vi "Simflight.vi"() -> ()   [LabVIEW 2014]
uses:
  subvis/state space loop data.ctl
  <vilib>/addons/Control Design/_Model Construction/Data Typedefs.llb/CD MIMO Time Response Data.ctl
  <vilib>/addons/Control Design/_Model Construction/Data Typedefs.llb/CD Plot Types Enum.ctl
  <vilib>/Utility/miscctls.llb/LV3DPointTypeDef.ctl
  <vilib>/Analysis/baseanly.llb/Real Outer Product.vi
  <vilib>/Analysis/Matrix/Numeric/Subtract/Subtract - RM,RM.vi
  <vilib>/addons/Control Design/_Model Construction/Model Creation.llb/Model Creation SubVI/cd_Create State Space Model.vi
  subvis/Data Xfer/subvis/Curcular Buffer Data History.vi
  <vilib>/Utility/inputDevices.llb/joystickAcquire.vi
  <vilib>/addons/Control Design/_Time Response Analysis/Time Response.llb/Time Response subVI/cd_Linear Simulation (State-Space).vi
  <vilib>/express/express arith-compare/Formula/XNode/ExpressFormulaBlockNode.xnode
  <vilib>/addons/Control Design/_Model Construction/NI_LinSys_Model Creation.lvlib
  <vilib>/addons/Control Design/_Time Response Analysis/NI_CD_Time Response.lvlib
  <vilib>/addons/Control Design/_Model Construction/NI_LinSys_Data Typedefs.lvlib
  subvis/attitude indicator/lv-attitudecontrol.lvlib
  <vilib>/Analysis/NI_AALBase.lvlib
  <vilib>/Analysis/Matrix/NI_Matrix.lvlib
panel:
  in  "device index":i32=2
  out "altitude 3":T1(graph)
  out "altitude 2":T1(graph)
  out "altitude":T1(graph)
  in  "elevator gain":dbl
  in  "aileron gain":dbl
  in  "rudder gain":dbl
  out "plot":T1(graph)
  in  "Aircraft":string="CDR"
  in  "Attitude Indicator":refnum<vi>(3d-picture)
  out "Airspeed (ft/s)":dbl(knob)=74.91519927978516 scale=0.0..80.0 scale format="%#.4f"
  out "motor (BHP)":cluster{dbl, dbl}(slide) scale=0.0..0.4
  out "ground track":cluster{"Time Stamp":dbl, "Data Value":dbl}[](graph)
  out "roll":dbl(slide) scale=-90.0..90.0
  out "pitch":dbl(slide) scale=-90.0..90.0
  out "rudder":cluster{dbl, dbl}(slide) scale=-25.0..25.0
  out "aileron":cluster{dbl, dbl}(slide) scale=-25.0..25.0
  out "elevator":cluster{dbl, dbl}(slide) scale=-35.0..35.0
  out "Heading":T2(graph)={"X"=[{"Y"=[21.620706805998168, 20.15124367946963, 12.465582235692763, 7.946576972490323, 11.656565240893995, 3.970903792227472, 5.440366929130449, 13.126028372052978, 19.003880895383112, 16.244982298473555, 16.832767550897515, 24.922937499080067, 24.33515224168201, 19.81289788882929, 13.93504536742159, 21.620706805998168], "Y"=[7.099604990531346, 5.077062500919932, 10.661022401488875, 5.291796067500631, 11.248807654089271, 16.832767550897515, 18.855310035128806, 13.271350139939326, 21.36152008350073, 25.220079209877188, 26.02909620777253, 20.151243679469633, 19.34222668734553, 20.773734831883043, 12.683564887248515, 7.099604990531346]}], "z"=[{"Y"=[15.0, 16.30733614, 17.60472267, 17.43107449, 17.60472267, 18.88228568, 20.13030215, 19.78828201, 20.13030215, 21.33927393, 22.5, 22.0, 22.5, 23.60364655, 24.64181415, 23.99902654, 24.64181415, 25.60660172, 26.49066665, 25.7246222, 26.49066665, 27.28728066, 27.99038106, 27.12435565, 27.99038106, 28.59461681, 29.09538931, 28.15569669, 29.09538931, 29.48888739, 29.7721163, 28.78730854, 29.7721163, 29.94292047, 30.0, 28.5, 30.0, 29.94292047, 29.7721163, 28.78730854, 29.7721163, 29.48888739, 29.09538931, 28.15569669, 29.09538931, 28.59461681, 27.99038106, 27.12435565, 27.99038106, 27.28728066, 26.49066665, 25.7246222, 26.49066665, 25.60660172, 24.64181415, 23.99902654, 24.64181415, 23.60364655, 22.5, 22.0, 22.5, 21.33927393, 20.13030215, 19.78828201, 20.13030215, 18.88228568, 17.60472267, 17.43107449, 17.60472267, 16.30733614, 15.0, 15.0, 15.0, 13.69266386, 12.39527733, 12.56892551, 12.39527733, 11.11771432, 9.86969785, 10.21171799, 9.86969785, 8.660726074, 7.5, 8.0, 7.5, 6.396353455, 5.358185855, 6.000973464, 5.358185855, 4.393398282, 3.509333353, 4.275377796, 3.509333353, 2.712719336, 2.009618943, 2.875644347, 2.009618943, 1.405383194, 0.904610688, 1.844303309, 0.904610688, 0.511112606, 0.227883705, 1.212691458, 0.227883705, 0.057079529, 0.0, 1.5, 0.0, 0.057079529, 0.227883705, 1.212691458, 0.227883705, 0.511112606, 0.904610688, 1.844303309, 0.904610688, 1.405383194, 2.009618943, 2.875644347, 2.009618943, 2.712719336, 3.509333353, 4.275377796, 3.509333353, 4.393398282, 5.358185855, 6.000973464, 5.358185855, 6.396353455, 7.5, 8.0, 7.5, 8.660726074, 9.86969785, 10.21171799, 9.86969785, 11.11771432, 12.39527733, 12.56892551, 12.39527733, 13.69266386, 15.0, 15.0], "Y"=[30.0, 29.94292047, 29.7721163, 28.78730854, 29.7721163, 29.48888739, 29.09538931, 28.15569669, 29.09538931, 28.59461681, 27.99038106, 27.12435565, 27.99038106, 27.28728066, 26.49066665, 25.7246222, 26.49066665, 25.60660172, 24.64181415, 23.99902654, 24.64181415, 23.60364655, 22.5, 22.0, 22.5, 21.33927393, 20.13030215, 19.78828201, 20.13030215, 18.88228568, 17.60472267, 17.43107449, 17.60472267, 16.30733614, 15.0, 15.0, 15.0, 13.69266386, 12.39527733, 12.56892551, 12.39527733, 11.11771432, 9.86969785, 10.21171799, 9.86969785, 8.660726074, 7.5, 8.0, 7.5, 6.396353455, 5.358185855, 6.000973464, 5.358185855, 4.393398282, 3.509333353, 4.275377796, 3.509333353, 2.712719336, 2.009618943, 2.875644347, 2.009618943, 1.405383194, 0.904610688, 1.844303309, 0.904610688, 0.511112606, 0.227883705, 1.212691458, 0.227883705, 0.057079529, 0.0, 1.5, 0.0, 0.057079529, 0.227883705, 1.212691458, 0.227883705, 0.511112606, 0.904610688, 1.844303309, 0.904610688, 1.405383194, 2.009618943, 2.875644347, 2.009618943, 2.712719336, 3.509333353, 4.275377796, 3.509333353, 4.393398282, 5.358185855, 6.000973464, 5.358185855, 6.396353455, 7.5, 8.0, 7.5, 8.660726074, 9.86969785, 10.21171799, 9.86969785, 11.11771432, 12.39527733, 12.56892551, 12.39527733, 13.69266386, 15.0, 15.0, 15.0, 16.30733614, 17.60472267, 17.43107449, 17.60472267, 18.88228568, 20.13030215, 19.78828201, 20.13030215, 21.33927393, 22.5, 22.0, 22.5, 23.60364655, 24.64181415, 23.99902654, 24.64181415, 25.60660172, 26.49066665, 25.7246222, 26.49066665, 27.28728066, 27.99038106, 27.12435565, 27.99038106, 28.59461681, 29.09538931, 28.15569669, 29.09538931, 29.48888739, 29.7721163, 28.78730854, 29.7721163, 29.94292047, 30.0, 28.5]}]}
  in  "visual":refnum<k7>(container) caption="3D 파라미터형 표면"
  in  "stop":bool
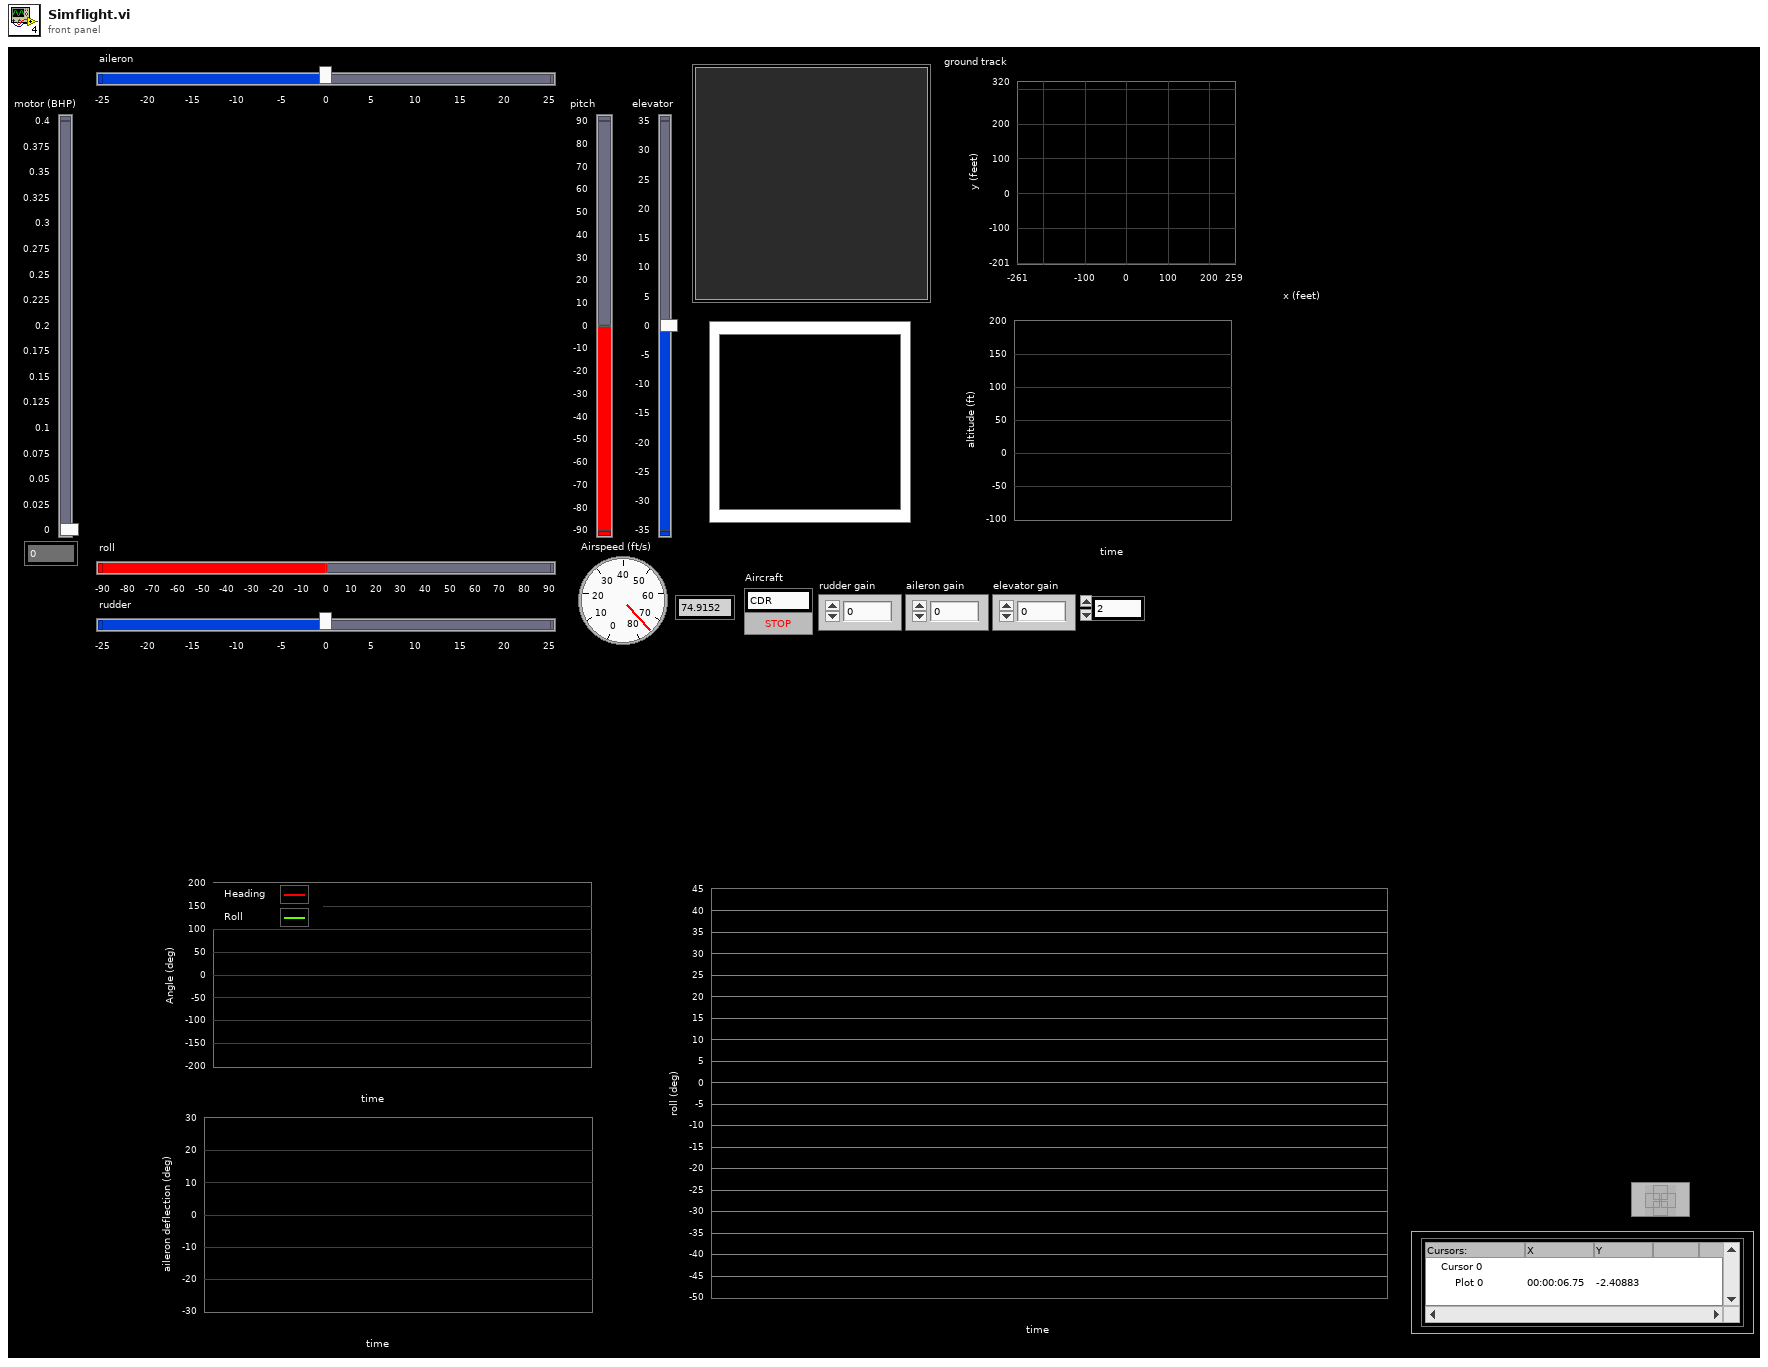
[diagram p1: front panel]
types:
  T1 = cluster{cluster{"Time Stamp":dbl, "Data Value":dbl}[]}[]
  T2 = cluster{"X":cluster{"Y":dbl[], "Y":dbl[]}[], "z":cluster{"Y":dbl[], "Y":dbl[]}[]}
  T3 = typedef "state space loop data.ctl" = cluster{"d_elevator (rad)":dbl, "d_rudder (rad)":dbl, "d_aileron (rad)":dbl, "d_motor (bhp)":dbl, "loop start (s)":dbl, "dT":dbl, "time now":dbl, "Sim Data":T4, "sim conditions":dbl[], "timestamp":dbl}
  T4 = typedef "NI_LinSys_Data Typedefs.lvlib/CD MIMO Time Response Data.ctl" = cluster{"Time":dbl[], "Outputs Data":dbl[][][], "States Data":dbl[][][], "plot type":T5}
  T5 = typedef "NI_LinSys_Data Typedefs.lvlib/CD Plot Types Enum.ctl" = enum16{"bode-magnitude", "bode-phase", "nichols", "nyquist", "singular values", "step", "impulse", "initial", "simulation", "nyquist with separation"}
  T6 = typedef "FlatEarth Inputs.ctl" = cluster{"a":dbl[][], "b":dbl[][], "c":dbl[][], "d":dbl[][], "du":dbl[][], "uIC":dbl[], "xIC":dbl[]}
  T7 = typedef "SIM INI.ctl" = cluster{"max_pwr":dbl, "max_rudder":dbl, "max_aileron":dbl, "max_elevator":dbl, "max_speed":dbl}
  T8 = typedef "NI_Matrix.lvlib/RealMatrix.ctl" = dbl[][]
  T9 = typedef "NI_LinSys_Model Typedefs.lvlib/CD State Space Model (MIMO).ctl" = cluster{"properties":T10, "A":dbl[][], "B":dbl[][], "C":dbl[][], "D":dbl[][], "StateNames":string[], "Transport Delay":dbl[][]}
  T10 = typedef "NI_LinSys_Model Typedefs.lvlib/CD General Elements.ctl" = cluster{"Model name":string, "Input names":string[], "Output names":string[], "Input Delays":dbl[], "Output Delays":dbl[], "Sampling Time":dbl, "Notes":string}
  T11 = typedef "lv-attitudecontrol.lvlib/AttitudeHandle.ctl" = cluster{"First Scene Object":refnum<vi>, "Drum":refnum<vi>, "Window":refnum<vi>, "Dial":refnum<vi>, "Scene Graph":refnum<vi>, "Last Drum Pitch":dbl, "Last Drum Roll ":dbl, "Last Dial Roll":dbl}
  T12 = cluster{"X axis":i32, "Y axis":i32, "Z axis":i32, "X axis rotation":i32, "Y axis rotation":i32, "Z axis rotation":i32, "U axis":i32, "V axis":i32}
  T13 = typedef "LV3DPointTypeDef.ctl" = cluster{"X":sgl, "Y":sgl, "Z":sgl}
  T14 = cluster{cluster{"Time Stamp":dbl, "Data Value":dbl}[]}
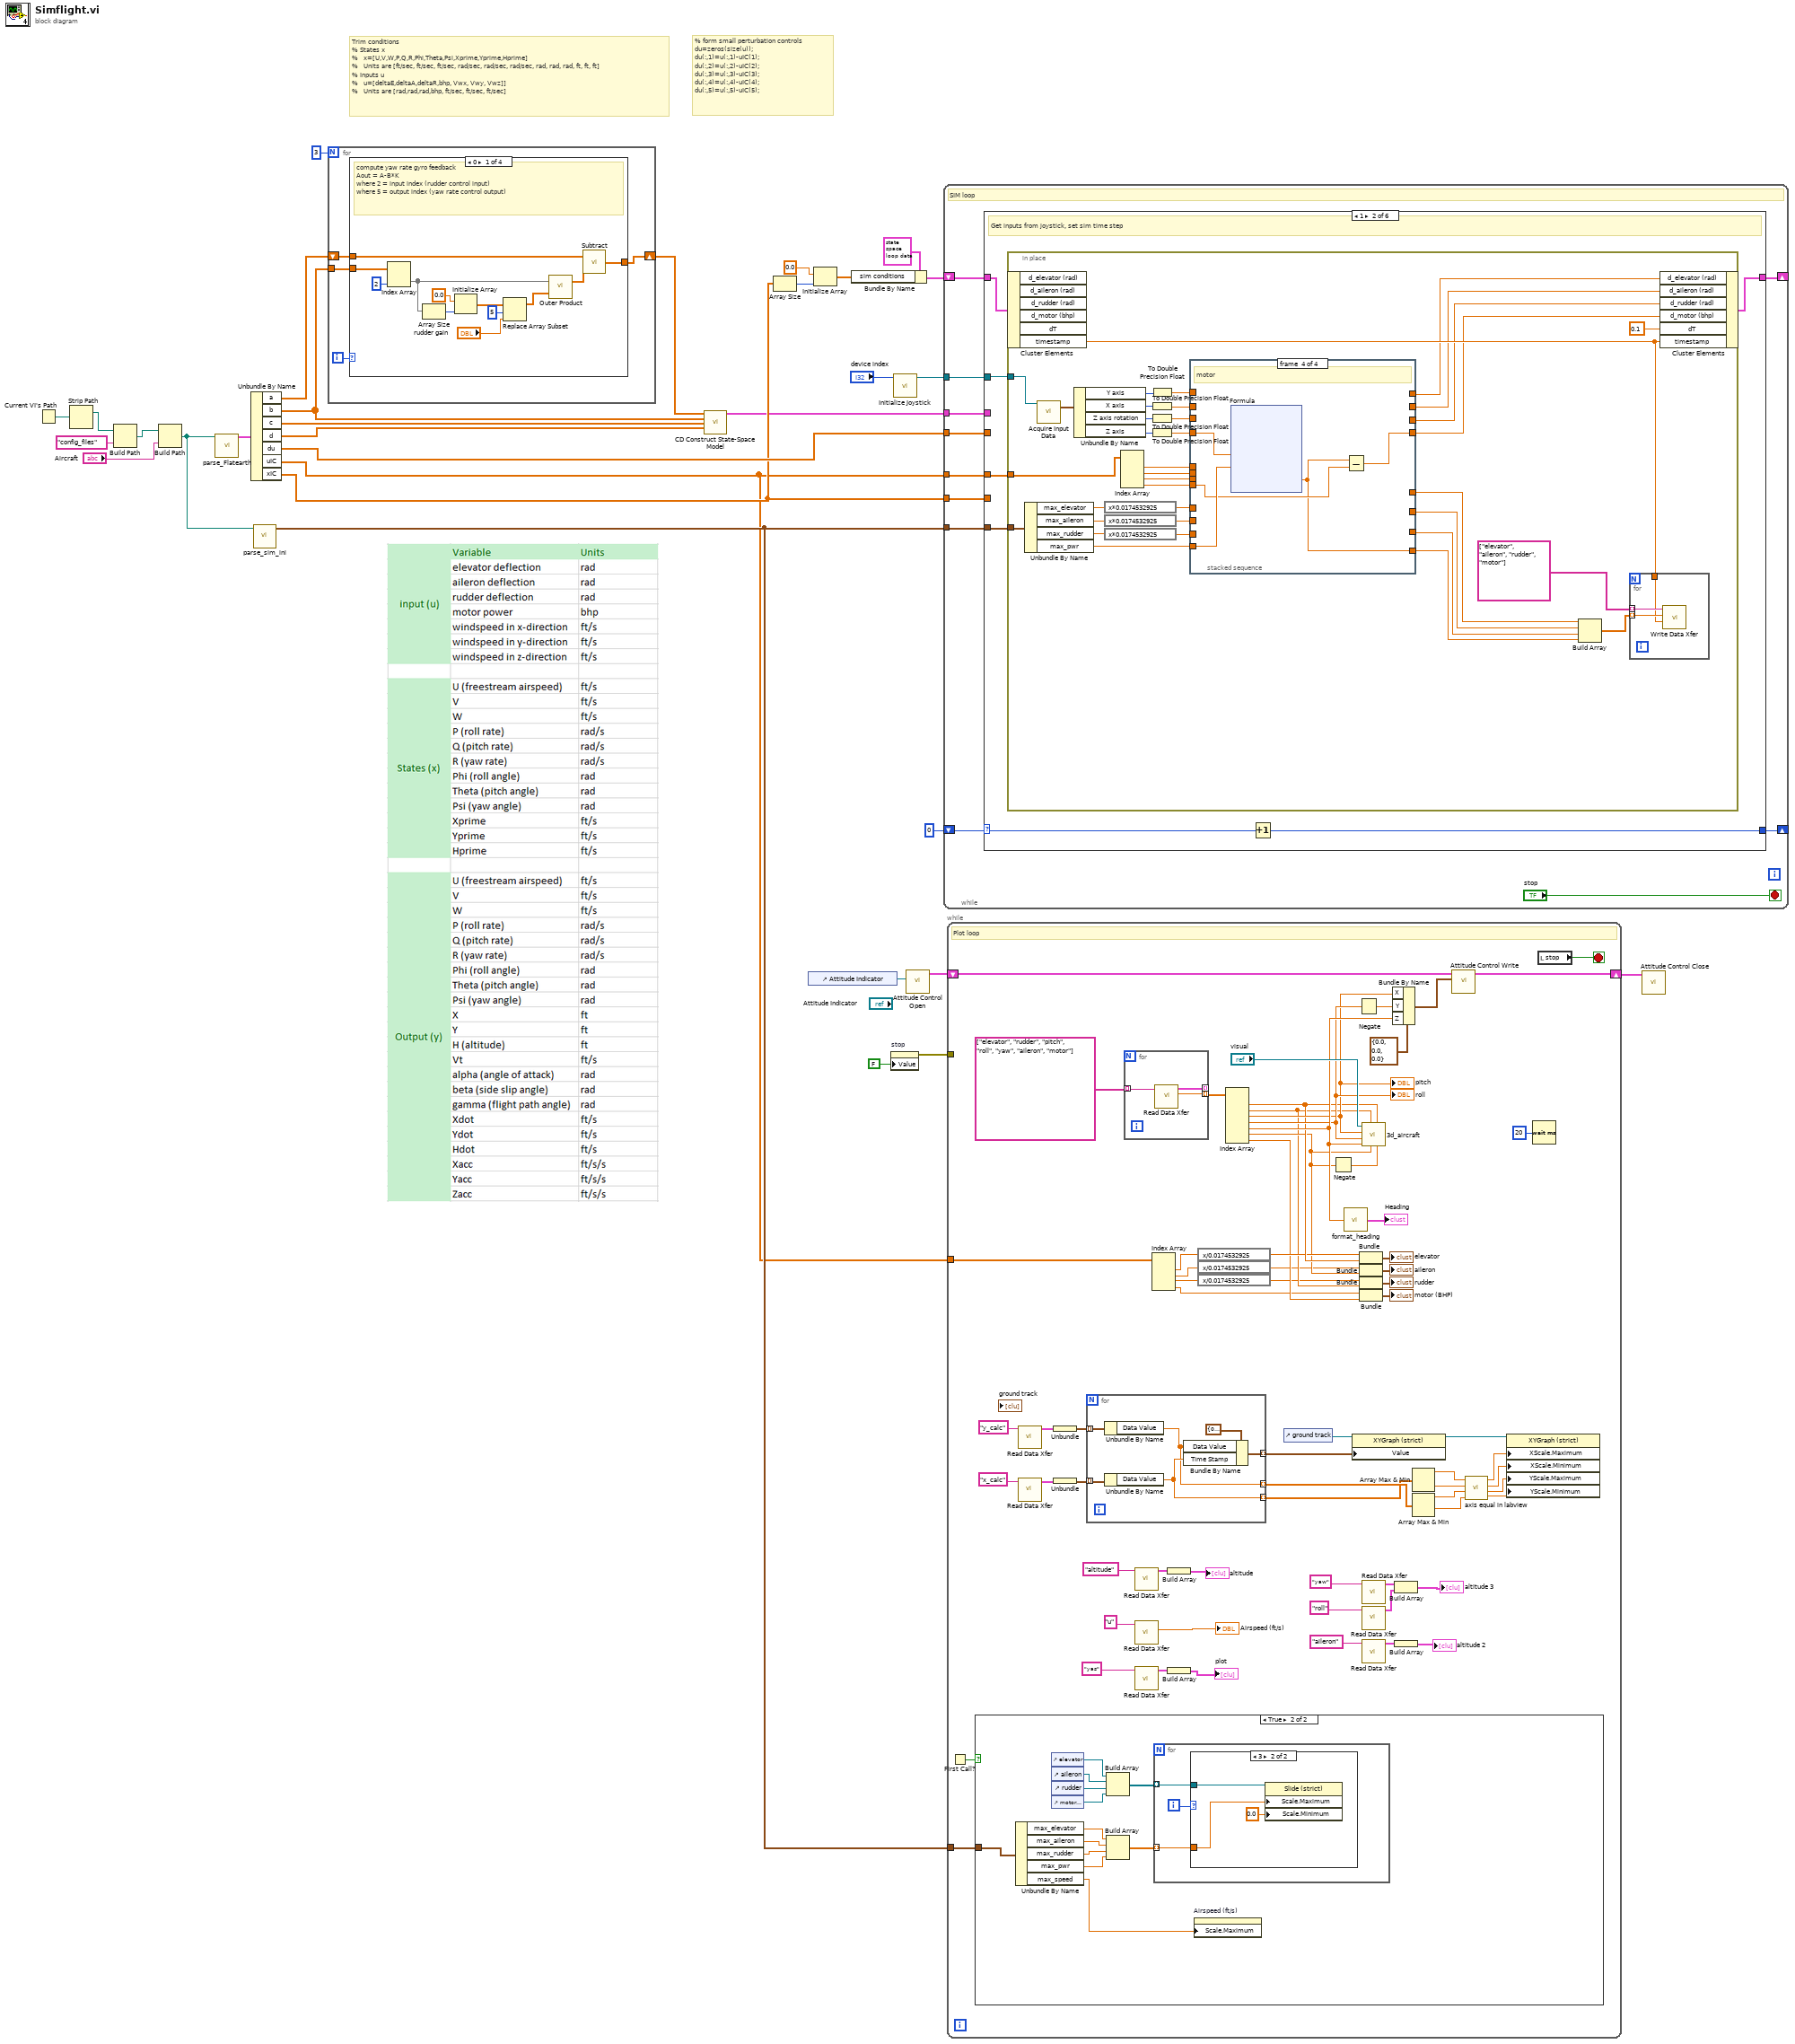
[diagram p0: block diagram]
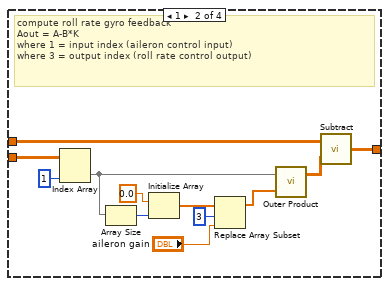
[diagram p2: hidden frame]
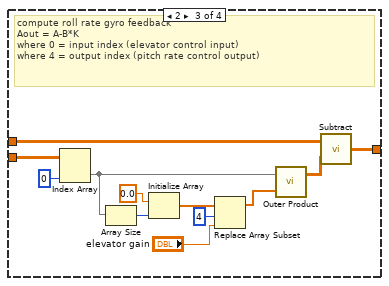
[diagram p3: hidden frame]
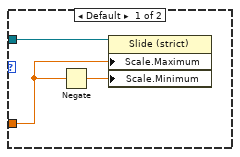
[diagram p6: hidden frame]
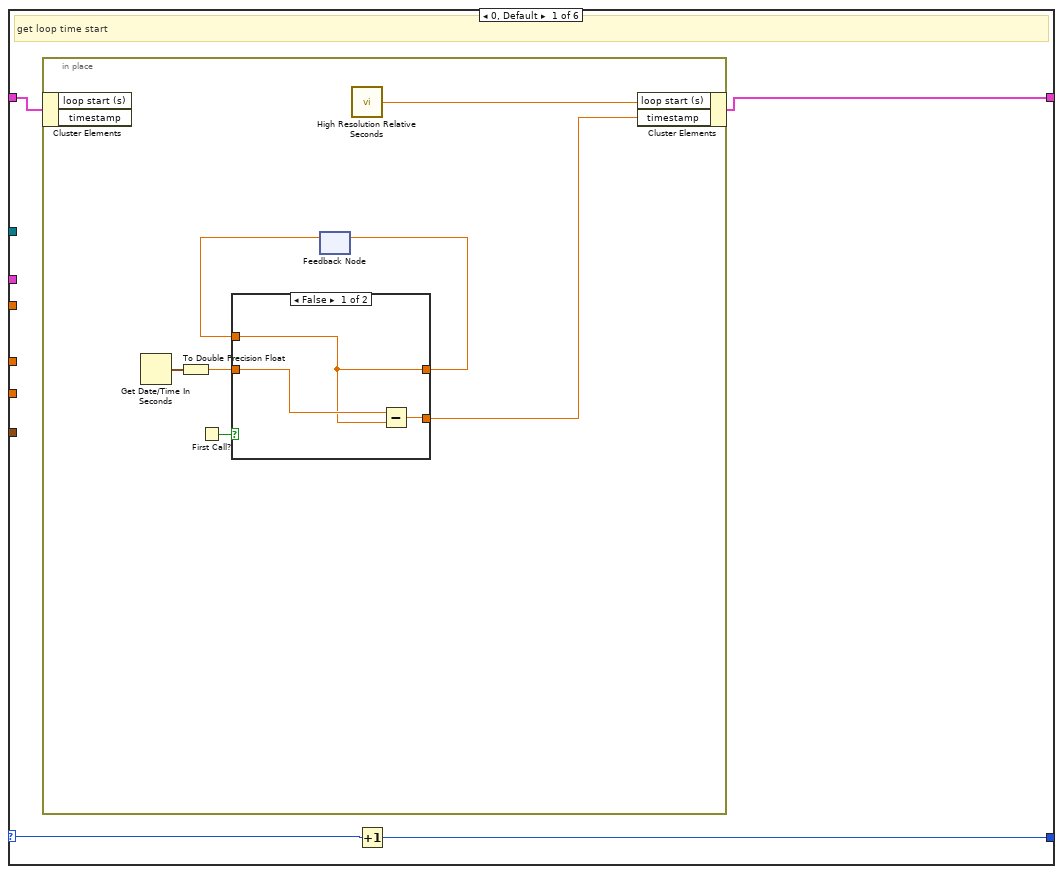
[diagram p7: hidden frame]
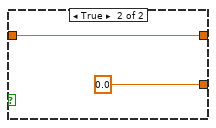
[diagram p8: hidden frame]
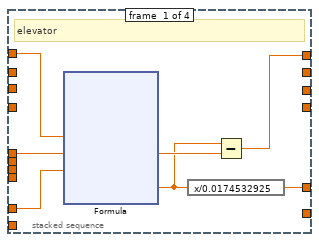
[diagram p9: hidden frame]
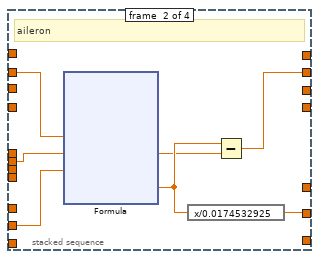
[diagram p10: hidden frame]
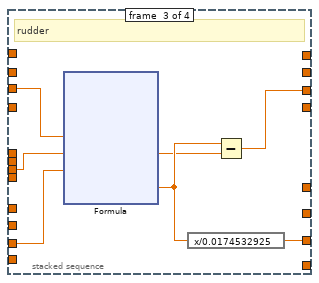
[diagram p11: hidden frame]
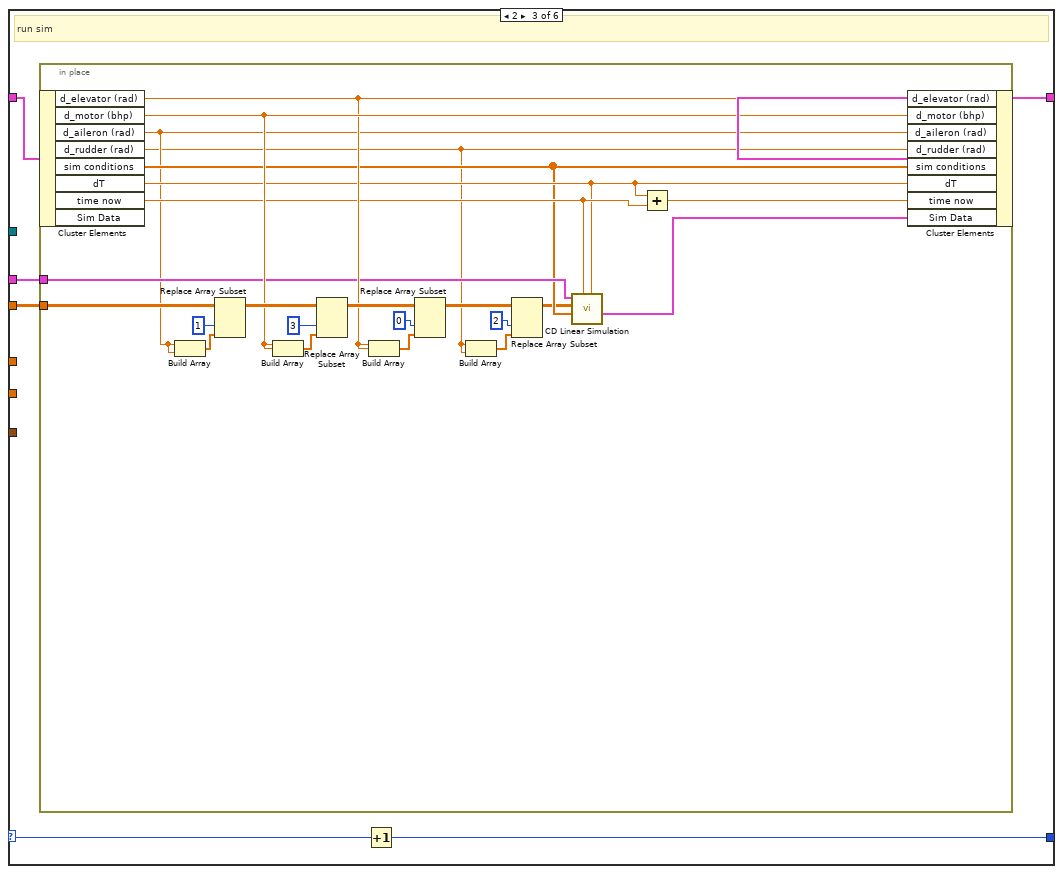
[diagram p12: hidden frame]
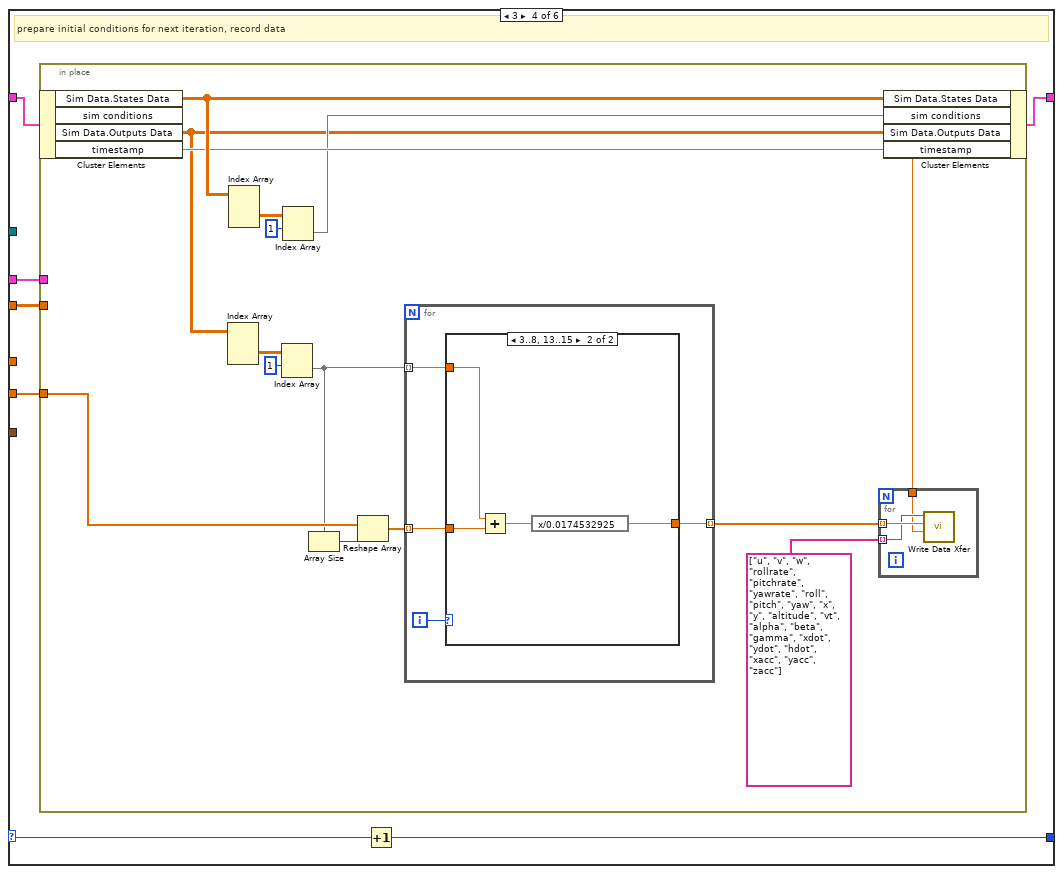
[diagram p13: hidden frame]
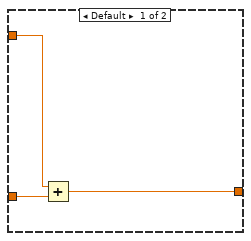
[diagram p14: hidden frame]
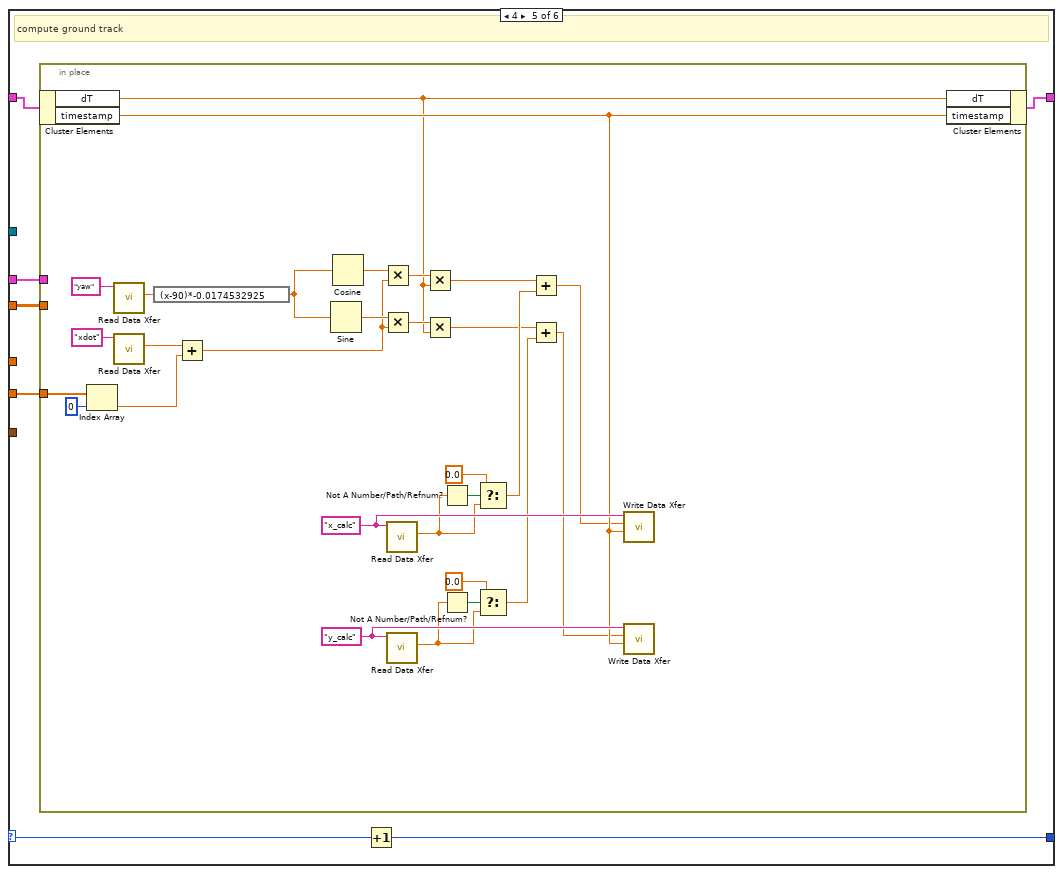
[diagram p15: hidden frame]
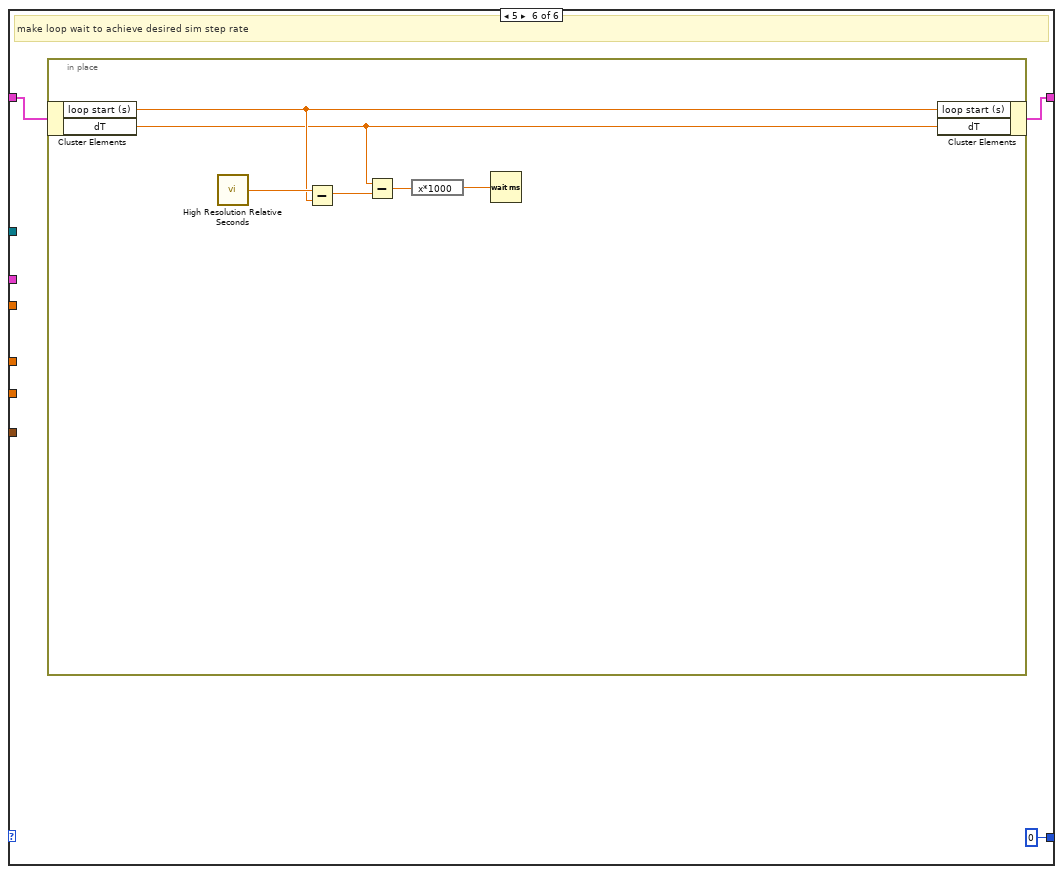
[diagram p16: hidden frame]
diagram:
  # "% form small perturbation controls\ndu=zeros(size(u));\ndu(:,1)=u(:,1)-uIC(1);\ndu(:,2)=u(:,2)-uIC(2);\ndu(:,3)=u(:,3)-uIC(3);\ndu(:,4)=u(:,4)-uIC(4);\ndu(:,5)=u(:,5)-uIC(5);"
  # "Trim conditions\n% States x\n%   x=[U,V,W,P,Q,R,Phi,Theta,Psi,Xprime,Yprime,Hprime]\n%   Units are [ft/sec, ft/sec, ft/sec, rad/sec, rad/sec, rad/sec, rad, rad, rad, ft, ft, ft]\n% Inputs u\n%   u=[deltaE,deltaA,deltaR,bhp, Vwx, Vwy, Vwz]]\n%   Units are [rad,rad,rad,bhp, ft/sec, ft/sec, ft/sec]"
  n1 = Current VI's Path() -> (path=w16:path)
  n2 = Strip Path(path=w16) -> (stripped path=w15:path)  [unwired: 1 out]
  n3 = Build Path(base path=w15, name or relative path="config_files") -> (appended path=w18:path)
  n4 = Build Path(base path=w18, name or relative path="Aircraft") -> (appended path=w7:path)
  n5 = call "parse_Flatearth.vi"("Parent path"=w7) -> ("FlatEarth Inputs"=w12:T6)  [unwired: 14 in]
  n6 = Unbundle By Name(w12) -> ("a"=w11:dbl[][], "b"=w10:dbl[][], "c"=w9:dbl[][], "d"=w8:dbl[][], "du"=w6:dbl[][], "uIC"=w3:dbl[], "xIC"=w5:dbl[])
  n7 = call "parse_sim_ini.vi"("Parent path"=w7) -> ("SIM INI"=w4:T7)  [unwired: 10 in]
  n8 = for {
    N: 3 -> [_]
    tunnel: w10 -> [w35]
    shift-right: [w33] -> w14
    shift-left: w11 -> [w34]
    i -> [w32]
    n9 = case shown="0" w32 {
      tunnel: w35 -> [w47 w59 w71 _]
      tunnel: w34 -> [w46 w58 w70 w72]
      tunnel: [w45 w57 w69 w72] -> w33
      frame 0 {
        # "compute yaw rate gyro feedback\nAout = A-B*K\nwhere 2 = input index (rudder control input)\nwhere 5 = output index (yaw rate control output)"
        n10 = Index Array(array=w47, index (col)=2 ("disabled index (col)")) -> (element=w40:dbl[])  [unwired: 1 in]
        n11 = Array Size(array=w40) -> (size(s)=w41:i32)
        n12 = Initialize Array(0.0, w41) -> (w39:dbl[])
        n13 = Replace Array Subset(array=w39, new element="rudder gain", index=5) -> (w36:dbl[])
        n14 = call-poly <vilib>:"Outer Product.vi"("Y Vector"=w36, "X Vector"=w40) -> ("Outer Product"=w43:T8)  [unwired: 1 out]
        n15 = call-poly <vilib>:"Subtract.vi"("Real Matrix B"=w43, "Real Matrix A"=w46) -> ("A - B"=w45:T8)
      }
      frame 1 {
        # "compute roll rate gyro feedback\nAout = A-B*K\nwhere 1 = input index (aileron control input)\nwhere 3 = output index (roll rate control output)"
        n16 = Index Array(array=w59, index (col)=1 ("disabled index (col)")) -> (element=w52:dbl[])  [unwired: 1 in]
        n17 = Array Size(array=w52) -> (size(s)=w53:i32)
        n18 = Initialize Array(0.0, w53) -> (w51:dbl[])
        n19 = Replace Array Subset(array=w51, new element="aileron gain", index=3) -> (w48:dbl[])
        n20 = call-poly <vilib>:"Outer Product.vi"("Y Vector"=w48, "X Vector"=w52) -> ("Outer Product"=w55:T8)  [unwired: 1 out]
        n21 = call-poly <vilib>:"Subtract.vi"("Real Matrix B"=w55, "Real Matrix A"=w58) -> ("A - B"=w57:T8)
      }
      frame 2 {
        # "compute roll rate gyro feedback\nAout = A-B*K\nwhere 0 = input index (elevator control input)\nwhere 4 = output index (pitch rate control output)"
        n22 = Index Array(array=w71, index (col)=0 ("disabled index (col)")) -> (element=w64:dbl[])  [unwired: 1 in]
        n23 = Array Size(array=w64) -> (size(s)=w65:i32)
        n24 = Initialize Array(0.0, w65) -> (w63:dbl[])
        n25 = Replace Array Subset(array=w63, new element="elevator gain", index=4) -> (w60:dbl[])
        n26 = call-poly <vilib>:"Outer Product.vi"("Y Vector"=w60, "X Vector"=w64) -> ("Outer Product"=w67:T8)  [unwired: 1 out]
        n27 = call-poly <vilib>:"Subtract.vi"("Real Matrix B"=w67, "Real Matrix A"=w70) -> ("A - B"=w69:T8)
      }
      frame Default {
        # "not used"
      }
    }
  }
  n28 = call-poly <vilib>:"CD Construct State-Space Model.vi"("A"=w14, "B"=w10, "C"=w9, "D"=w8) -> ("State-Space Model"=w2:T9)  [unwired: 10 in, 1 out]
  n29 = Array Size(array=w5) -> (size(s)=w25:i32)
  n30 = control-ref of="Attitude Indicator"() -> (w22:refnum<vi>)
  n31 = Initialize Array(0.0, w25) -> (w23:dbl[])
  n32 = Bundle By Name(cluster=T3 {"d_elevator (rad)"=0.0, "d_rudder (rad)"=0.0, "d_aileron (rad)"=0.0, "d_motor (bhp)"=0.0, "loop start (s)"=0.0, "dT"=0.0, "time now"=0.0, "Sim Data"={"Time"=[], "Outputs Data"=[], "States Data"=[], "plot type"=enum."step"}, "sim conditions"=[], "timestamp"=0.0}, "sim conditions"=w23) -> (w28:T3)
  n33 = property on="stop" class="Bool (strict)"("Value"=FALSE ("stop")) -> (error out=w26:errorcluster)  [unwired: 2 in, 1 out]
  n34 = call <vilib>:"Initialize Joystick.vi"("device index"="device index") -> ("device ID"=w31:refnum<k1>)  [unwired: 9 in, 1 out]
  n35 = call "Attitude Control Open.vi"("Scene Graph"=w22) -> ("Attitude Control Handle"=w21:T11)  [unwired: 9 in, 1 out]
  n36 = while {
    shift-right: [w82] -> _
    shift-left: w28 -> [w83]
    tunnel: w31 -> [w81]
    shift-right: [w80] -> _
    shift-left: 0 -> [w79]
    tunnel: w2 -> [w77]
    tunnel: w6 -> [w76]
    tunnel: w3 -> [w75]
    tunnel: w5 -> [w74]
    tunnel: w4 -> [w73]
    stop <- "stop" stop-if-true
    # "SIM loop"
    n37 = case shown="1" w79 {
      tunnel: w83 -> [w85 w105 w219 w249 w284 w315]
      tunnel: [w84 w104 w218 w248 w283 w314] -> w82
      tunnel: w81 -> [_ w106 _ _ _ _]
      selector: w79 -> [w87 w103 w217 w247 w282 _]
      tunnel: [w86 w102 w216 w246 w281 0] -> w80
      tunnel: w77 -> [_ _ w214 w244 w279 _]
      tunnel: w76 -> [_ _ w215 w245 w280 _]
      tunnel: w75 -> [_ w100 _ _ _ _]
      tunnel: w74 -> [_ _ _ w243 w278 _]
      tunnel: w73 -> [_ w101 _ _ _ _]
      frame 0, Default {
        # "get loop time start"
        n38 = in-place {
          n39 = in-place-cluster #1(w85) -> ()  [unwired: 2 out]
          n40 = Get Date/Time In Seconds() -> (seconds since 1Jan1904=w93:timestamp)
          n41 = To Double Precision Float(number=w93) -> (double precision float=w91:dbl)
          n42 = First Call?() -> (First Call?: T/F=w92:bool)
          n43 = feedback #2() -> (w89:dbl)  [unwired: 1 in]
          n44 = case shown="False" w92 {
            tunnel: w91 -> [w96 w99]
            tunnel: [w95 w99] -> w90
            tunnel: w89 -> [w95 _]
            tunnel: [w97 0.0] -> w88
            frame False {
              n45 = Subtract(x=w96, y=w95) -> (x-y=w97:dbl)
            }
            frame True {
            }
          }
          n46 = feedback-in #2(w90) -> ()
          n47 = call <vilib>:"High Resolution Relative Seconds.vi"() -> ("relative seconds"=w94:dbl)
          n48 = in-place-cluster #1("loop start (s)"=w94, "timestamp"=w88) -> (w84:T3)
        }
        n49 = Increment(x=w87) -> (x+1=w86:i32)
      }
      frame 1 {
        # "Get inputs from joystick, set sim time step"
        n50 = in-place {
          in-place-border: w106 -> [w140]
          in-place-border: w101 -> [w133]
          in-place-border: w100 -> [w128]
          n51 = in-place-cluster #3(w105) -> ("timestamp"=w135:dbl)  [unwired: 5 out]
          n52 = Unbundle By Name(w133) -> ("max_elevator"=w123:dbl, "max_aileron"=w121:dbl, "max_rudder"=w122:dbl, "max_pwr"=w117:dbl)
          n53 = call-poly <vilib>:"Acquire Input Data.vi"("device ID"=w140) -> ("axis info"=w139:T12)  [unwired: 14 in, 4 out]
          n54 = Unbundle By Name(w139) -> ("Y axis"=w141:i32, "X axis"=w138:i32, "Z axis rotation"=w137:i32, "Z axis"=w134:i32)
          n55 = expression code="x*0.0174532925"(w123) -> (w120:dbl)
          n56 = expression code="x*0.0174532925"(w121) -> (w119:dbl)
          n57 = expression code="x*0.0174532925"(w122) -> (w118:dbl)
          n58 = Index Array(array=w128) -> (element #1=w127:dbl, element #2=w126:dbl, element #3=w125:dbl, element #4=w124:dbl)  [unwired: 4 in]
          n59 = To Double Precision Float(number=w138) -> (double precision float=w131:dbl)
          n60 = To Double Precision Float(number=w137) -> (double precision float=w130:dbl)
          n61 = To Double Precision Float(number=w134) -> (double precision float=w129:dbl)
          n62 = To Double Precision Float(number=w141) -> (double precision float=w132:dbl)
          n63 = stacked-sequence {
            tunnel: w132 -> [w147 _ _ _]
            tunnel: w131 -> [_ w165 _ _]
            tunnel: w130 -> [_ _ w183 _]
            tunnel: w129 -> [_ _ _ w200]
            tunnel: w120 -> [w146 _ _ _]
            tunnel: w127 -> [w145 _ _ _]
            tunnel: w126 -> [_ w161 _ _]
            tunnel: w125 -> [_ _ w180 _]
            tunnel: w124 -> [_ _ _ w198]
            tunnel: w119 -> [_ w164 _ _]
            tunnel: w118 -> [_ _ w182 _]
            tunnel: w117 -> [_ _ _ w199]
            tunnel: [w143 _ _ _] -> w109
            tunnel: [_ w162 _ _] -> w108
            tunnel: [_ _ w178 _] -> w107
            tunnel: [_ _ _ w197] -> w114
            tunnel: [w144 _ _ _] -> w113
            tunnel: [_ w160 _ _] -> w112
            tunnel: [_ _ w179 _] -> w111
            tunnel: [_ _ _ w196] -> w110
            frame #0 {
              # "elevator"
              n64 = xnode "Formula"("input"=w147, "Trim"=w145, "Max"=w146) -> ("Result"=w142:dbl)  [unwired: 1 in, 1 out]
              n65 = expression code="x/0.0174532925"(w142) -> (w143:dbl)
              n66 = Subtract(x=w142, y=w145) -> (x-y=w144:dbl)
            }
            frame #1 {
              # "aileron"
              n67 = xnode "Formula"("input"=w165, "Trim"=w161, "Max"=w164) -> ("Result"=w163:dbl)  [unwired: 1 in, 1 out]
              n68 = expression code="x/0.0174532925"(w163) -> (w162:dbl)
              n69 = Subtract(x=w163, y=w161) -> (x-y=w160:dbl)
            }
            frame #2 {
              # "rudder"
              n70 = xnode "Formula"("input"=w183, "Trim"=w180, "Max"=w182) -> ("Result"=w181:dbl)  [unwired: 1 in, 1 out]
              n71 = expression code="x/0.0174532925"(w181) -> (w178:dbl)
              n72 = Subtract(x=w181, y=w180) -> (x-y=w179:dbl)
            }
            frame #3 {
              # "motor"
              n73 = xnode "Formula"("input"=w200, "Max"=w199) -> ("Result"=w197:dbl)  [unwired: 1 in, 1 out]
              n74 = Subtract(x=w197, y=w198) -> (x-y=w196:dbl)
            }
          }
          n75 = Build Array(w109, w108, w107, w114) -> (w115:dbl[])
          n76 = for {
            tunnel: w115 -> [w213] mode=indexing
            tunnel: string[] ["elevator", "aileron", "rudder", "motor"] -> [w212] mode=indexing
            tunnel: w135 -> [w211]
            n77 = call "Write Data Xfer.vi"("Time Stamp"=w211, "Data Value"=w213, "Device Name"=w212) -> ()  [unwired: 8 in, 1 out]
          }
          n78 = in-place-cluster #3("d_elevator (rad)"=w113, "d_aileron (rad)"=w112, "d_rudder (rad)"=w111, "d_motor (bhp)"=w110, "dT"=0.1, "timestamp"=w135) -> (w104:T3)
        }
        n79 = Increment(x=w103) -> (x+1=w102:i32)
      }
      frame 2 {
        # "run sim"
        n80 = in-place {
          in-place-border: w215 -> [w237]
          in-place-border: w214 -> [w231]
          n81 = in-place-cluster #4(w219) -> ("d_elevator (rad)"=w232:dbl, "d_motor (bhp)"=w234:dbl, "d_aileron (rad)"=w225:dbl, "d_rudder (rad)"=w220:dbl, "sim conditions"=w226:dbl[], "dT"=w229:dbl, "time now"=w230:dbl)  [unwired: 1 out]
          n82 = Build Array(w225, w225) -> (w236:dbl[])
          n83 = Replace Array Subset(array=w237, new element=w236, index (col)=1 ("disabled index (col)")) -> (w242:dbl[][])  [unwired: 1 in]
          n84 = Build Array(w234, w234) -> (w235:dbl[])
          n85 = Replace Array Subset(array=w242, new element=w235, index (col)=3 ("disabled index (col)")) -> (w239:dbl[][])  [unwired: 1 in]
          n86 = Build Array(w232, w232) -> (w233:dbl[])
          n87 = Replace Array Subset(array=w239, new element=w233, index (col)=0 ("index")) -> (w222:dbl[][])  [unwired: 1 in]
          n88 = Build Array(w220, w220) -> (w224:dbl[])
          n89 = Replace Array Subset(array=w222, new element=w224, index (col)=2 ("index")) -> (w221:dbl[][])  [unwired: 1 in]
          n90 = call-poly <vilib>:"CD Linear Simulation.vi"("Delta t"=w229, "Initial Time"=w230, "Initial Conditions"=w226, "Inputs"=w221, "State-Space Model"=w231) -> ("Simulation Data"=w227:T4)  [unwired: 3 in, 3 out]
          n91 = Add(x=w229, y=w230) -> (x+y=w228:dbl)
          n92 = in-place-cluster #4("d_elevator (rad)"=w232, "d_motor (bhp)"=w234, "d_aileron (rad)"=w225, "d_rudder (rad)"=w220, "sim conditions"=w226, "dT"=w229, "time now"=w228, "Sim Data"=w227) -> (w218:T3)
        }
        n93 = Increment(x=w217) -> (x+1=w216:i32)
      }
      frame 3 {
        # "prepare initial conditions for next iteration, record data"
        n94 = in-place {
          in-place-border: w245 -> [_]
          in-place-border: w244 -> [_]
          in-place-border: w243 -> [w252]
          n95 = in-place-cluster #5(w249) -> ("Sim Data.States Data"=w261:dbl[][][], "Sim Data.Outputs Data"=w255:dbl[][][], "timestamp"=w260:dbl)  [unwired: 1 out]
          n96 = Index Array(array=w255) -> (element=w257:dbl[][])  [unwired: 3 in]
          n97 = Index Array(array=w261) -> (element=w262:dbl[][])  [unwired: 3 in]
          n98 = Index Array(array=w257, index (row)=1) -> (element=w250:dbl[])  [unwired: 1 in]
          n99 = Index Array(array=w262, index (row)=1) -> (element=w259:dbl[])  [unwired: 1 in]
          n100 = Array Size(array=w250) -> (size(s)=w251:i32)
          n101 = Reshape Array(w252, w251) -> (w253:dbl[])
          n102 = for {
            tunnel: w250 -> [w266] mode=indexing
            tunnel: w253 -> [w265] mode=indexing
            tunnel: [w264] -> w258 mode=indexing
            i -> [w267]
            n103 = case shown="3..8, 13..15" w267 {
              tunnel: w266 -> [w269 w273]
              tunnel: w265 -> [w270 w274]
              tunnel: [w268 w271] -> w264
              frame Default {
                n104 = Add(x=w269, y=w270) -> (x+y=w268:dbl)
              }
              frame 3..8, 13..15 {
                n105 = Add(x=w273, y=w274) -> (x+y=w272:dbl)
                n106 = expression code="x/0.0174532925"(w272) -> (w271:dbl)
              }
            }
          }
          n107 = for {
            tunnel: w258 -> [w277] mode=indexing
            tunnel: string[] ["u", "v", "w", "rollrate", "pitchrate", "yawrate", "roll", "pitch", "yaw", "x", "y", "altitude", "vt", "alpha", "beta", "gamma", "xdot", "ydot", "hdot", "xacc", "yacc", "zacc"] -> [w276] mode=indexing
            tunnel: w260 -> [w275]
            n108 = call "Write Data Xfer.vi"("Time Stamp"=w275, "Data Value"=w277, "Device Name"=w276) -> ()  [unwired: 8 in, 1 out]
          }
          n109 = in-place-cluster #5("Sim Data.States Data"=w261, "sim conditions"=w259, "Sim Data.Outputs Data"=w255, "timestamp"=w260) -> (w248:T3)
        }
        n110 = Increment(x=w247) -> (x+1=w246:i32)
      }
      frame 4 {
        # "compute ground track"
        n111 = in-place {
          in-place-border: w280 -> [_]
          in-place-border: w279 -> [_]
          in-place-border: w278 -> [w302]
          w311 = "x_calc"
          w312 = "y_calc"
          n112 = in-place-cluster #6(w284) -> ("dT"=w292:dbl, "timestamp"=w310:dbl)
          n113 = Index Array(array=w302, index=0) -> (element=w301:dbl)
          n114 = call "Read Data Xfer.vi"("Device Name"="yaw") -> ("Latest Value"=w298:dbl)  [unwired: 7 in, 3 out]
          n115 = call "Read Data Xfer.vi"("Device Name"="xdot") -> ("Latest Value"=w300:dbl)  [unwired: 7 in, 3 out]
          n116 = expression code="(x-90)*-0.0174532925"(w298) -> (w297:dbl)
          n117 = Add(x=w300, y=w301) -> (x+y=w285:dbl)
          n118 = Sine(x=w297) -> (sin(x)=w295:dbl)
          n119 = Cosine(x=w297) -> (cos(x)=w296:dbl)
          n120 = Multiply(x=w296, y=w285) -> (x*y=w294:dbl)
          n121 = Multiply(x=w295, y=w285) -> (x*y=w293:dbl)
          n122 = call "Read Data Xfer.vi"("Device Name"=w311) -> ("Latest Value"=w307:dbl)  [unwired: 7 in, 3 out]
          n123 = call "Read Data Xfer.vi"("Device Name"=w312) -> ("Latest Value"=w304:dbl)  [unwired: 7 in, 3 out]
          n124 = Multiply(x=w294, y=w292) -> (x*y=w291:dbl)
          n125 = Multiply(x=w293, y=w292) -> (x*y=w288:dbl)
          n126 = Not A Number/Path/Refnum?(number/path/refnum=w307) -> (NaN/Path/Refnum?=w309:bool)
          n127 = Not A Number/Path/Refnum?(number/path/refnum=w304) -> (NaN/Path/Refnum?=w305:bool)
          n128 = Select(t=0.0, s=w309, f=w307) -> (s? t:f=w290:dbl)
          n129 = Select(t=0.0, s=w305, f=w304) -> (s? t:f=w287:dbl)
          n130 = Add(x=w291, y=w290) -> (x+y=w289:dbl)
          n131 = Add(x=w288, y=w287) -> (x+y=w286:dbl)
          n132 = call "Write Data Xfer.vi"("Time Stamp"=w310, "Data Value"=w289, "Device Name"=w311) -> ()  [unwired: 8 in, 1 out]
          n133 = call "Write Data Xfer.vi"("Time Stamp"=w310, "Data Value"=w286, "Device Name"=w312) -> ()  [unwired: 8 in, 1 out]
          n134 = in-place-cluster #6("dT"=w292, "timestamp"=w310) -> (w283:T3)
        }
        n135 = Increment(x=w282) -> (x+1=w281:i32)
      }
      frame 5 {
        # "make loop wait to achieve desired sim step rate"
        n136 = in-place {
          n137 = in-place-cluster #7(w315) -> ("loop start (s)"=w320:dbl, "dT"=w319:dbl)
          n138 = call <vilib>:"High Resolution Relative Seconds.vi"() -> ("relative seconds"=w322:dbl)
          n139 = Subtract(x=w322, y=w320) -> (x-y=w321:dbl)
          n140 = Subtract(x=w319, y=w321) -> (x-y=w317:dbl)
          n141 = expression code="x*1000"(w317) -> (w318:dbl)
          n142 = Wait (ms)(milliseconds to wait=w318) -> ()  [unwired: 1 out]
          n143 = in-place-cluster #7("loop start (s)"=w320, "dT"=w319) -> (w314:T3)
        }
      }
    }
  }
  n144 = while {
    tunnel: w26 -> [_]
    shift-right: [w369] -> w20
    shift-left: w21 -> [w371]
    tunnel: w4 -> [w340]
    tunnel: w3 -> [w338]
    stop <- w390 stop-if-true
    # "Plot loop"
    n145 = First Call?() -> (First Call?: T/F=w339:bool)
    n146 = case shown="True" w339 {
      tunnel: w340 -> [_ w402]
      frame False {
      }
      frame True {
        n147 = Unbundle By Name(w402) -> ("max_elevator"=w401:dbl, "max_aileron"=w400:dbl, "max_rudder"=w398:dbl, "max_pwr"=w399:dbl, "max_speed"=w391:dbl)
        n148 = control-ref of="elevator"() -> (w392:refnum<vi>)
        n149 = control-ref of="aileron"() -> (w393:refnum<vi>)
        n150 = control-ref of="rudder"() -> (w394:refnum<vi>)
        n151 = control-ref of="motor (BHP)"() -> (w395:refnum<vi>)
        n152 = Build Array(w392, w393, w394, w395) -> (w397:refnum<vi>[])
        n153 = Build Array(w401, w400, w398, w399) -> (w396:dbl[])
        n154 = for {
          tunnel: w397 -> [w405] mode=indexing
          tunnel: w396 -> [w404] mode=indexing
          i -> [w403]
          n155 = case shown="3" w403 {
            tunnel: w405 -> [w408 w411]
            tunnel: w404 -> [w406 w410]
            frame Default {
              n156 = Negate(x=w406) -> (-x=w407:dbl)
              n157 = property class="Slide (strict)"(reference=w408, "Scale.Maximum"=w406, "Scale.Minimum"=w407) -> ()  [unwired: 1 in, 2 out]
            }
            frame 3 {
              n158 = property class="Slide (strict)"(reference=w411, "Scale.Maximum"=w410, "Scale.Minimum"=0.0 ("Scale.Range:Minimum")) -> ()  [unwired: 1 in, 2 out]
            }
          }
        }
        n159 = property on="Airspeed (ft/s)" class="Knob (strict)"("Scale.Maximum"=w391) -> ()  [unwired: 2 in, 2 out]
      }
    }
    n160 = call "Read Data Xfer.vi"("Device Name"="y_calc") -> ("Truncated Data History"=w381:T14)  [unwired: 7 in, 3 out]
    n161 = call "Read Data Xfer.vi"("Device Name"="x_calc") -> ("Truncated Data History"=w379:T14)  [unwired: 7 in, 3 out]
    n162 = Unbundle(w381) -> (w380:cluster{"Time Stamp":dbl, "Data Value":dbl}[])
    n163 = Unbundle(w379) -> (w378:cluster{"Time Stamp":dbl, "Data Value":dbl}[])
    n164 = for {
      tunnel: w380 -> [w417] mode=indexing
      tunnel: w378 -> [w416] mode=indexing
      tunnel: [w414] -> w364 mode=indexing
      tunnel: [w413] -> w357 mode=indexing
      tunnel: [w412] -> w358 mode=indexing
      n165 = Unbundle By Name(w417) -> ("Data Value"=w412:dbl)
      n166 = Unbundle By Name(w416) -> ("Data Value"=w413:dbl)
      n167 = Bundle By Name(cluster=cluster{"Time Stamp":dbl, "Data Value":dbl} {"Time Stamp"=0.0, "Data Value"=0.0}, "Data Value"=w412, "Time Stamp"=w413) -> (w414:cluster{"Time Stamp":dbl, "Data Value":dbl})
    }
    n168 = for {
      tunnel: string[] ["elevator", "rudder", "pitch", "roll", "yaw", "aileron", "motor"] -> [w420] mode=indexing
      tunnel: [w419] -> w386 mode=indexing
      tunnel: [w418] -> _ mode=indexing
      n169 = call "Read Data Xfer.vi"("Device Name"=w420) -> ("Latest Value"=w419:dbl, "Truncated Data History"=w418:T14)  [unwired: 7 in, 2 out]
    }
    n170 = call "Read Data Xfer.vi"("Device Name"="altitude") -> ("Truncated Data History"=w376:T14)  [unwired: 7 in, 3 out]
    n171 = call "Read Data Xfer.vi"("Device Name"="u") -> ("Latest Value"=→"Airspeed (ft/s)":dbl)  [unwired: 7 in, 3 out]
    n172 = call "Read Data Xfer.vi"("Device Name"="yas") -> ("Truncated Data History"=w351:T14)  [unwired: 7 in, 3 out]
    n173 = Index Array(array=w338) -> (element #1=w337:dbl, element #2=w336:dbl, element #3=w335:dbl, element #4=w325:dbl)  [unwired: 4 in]
    n174 = Build Array(w376) -> (→"altitude":T1)
    n175 = Build Array(w351) -> (→"plot":T1)
    n176 = expression code="x/0.0174532925"(w337) -> (w332:dbl)
    n177 = expression code="x/0.0174532925"(w336) -> (w327:dbl)
    n178 = expression code="x/0.0174532925"(w335) -> (w326:dbl)
    n179 = Index Array(array=w386) -> (element #1=w333:dbl, element #2=w330:dbl, element #3=w366:dbl, element #4=w367:dbl, element #5=w372:dbl, element #6=w331:dbl, element #7=w329:dbl)  [unwired: 7 in]
    "roll" <- w367
    "pitch" <- w366
    n180 = control-ref of="ground track"() -> (w365:refnum<vi>)
    n181 = Negate(x=w331) -> (-x=w385:dbl)
    n182 = call "format_heading.vi"("Heading (deg)"=w372) -> ("heading (formatted)"=→"Heading":T2)
    n183 = property class="XYGraph (strict)"(reference=w365, "Value"=w364) -> (reference out=w363:refnum<vi>)  [unwired: 1 in, 1 out]
    n184 = Negate(x=w367) -> (-x=w368:dbl)
    n185 = Bundle(w332, "Latest Value"=w333) -> (→"elevator":cluster{dbl, "Latest Value":dbl})  [unwired: 1 in]
    n186 = Bundle(w327, "Latest Value"=w331) -> (→"aileron":cluster{dbl, "Latest Value":dbl})  [unwired: 1 in]
    n187 = Bundle(w326, "Latest Value"=w330) -> (→"rudder":cluster{dbl, "Latest Value":dbl})  [unwired: 1 in]
    n188 = Bundle(w325, "Latest Value"=w329) -> (→"motor (BHP)":cluster{dbl, "Latest Value":dbl})  [unwired: 1 in]
    n189 = call "3d_aircraft.vi"("RH Aileron"=w385, "Elevator"=w333, "LH Aileron"=w331, "Rudder"=w330, "Heading (deg)"=w372, "Roll (deg)"=w367, "Pitch (deg)"=w366, "visual"="visual") -> ()  [unwired: 4 in]
    n190 = call "Read Data Xfer.vi"("Device Name"="yaw") -> ("Truncated Data History"=w347:T14)  [unwired: 7 in, 3 out]
    n191 = call "Read Data Xfer.vi"("Device Name"="roll") -> ("Truncated Data History"=w341:T14)  [unwired: 7 in, 3 out]
    n192 = call "Read Data Xfer.vi"("Device Name"="aileron") -> ("Truncated Data History"=w346:T14)  [unwired: 7 in, 3 out]
    n193 = Bundle By Name(cluster=T13 {"X"=0.0, "Y"=0.0, "Z"=0.0} ("Control 1"), "X"=w366, "Y"=w368, "Z"=w372) -> (w370:T13)
    n194 = Build Array(w347, w341) -> (→"altitude 3":T1)
    n195 = Build Array(w346) -> (→"altitude 2":T1)
    n196 = Array Max & Min(array=w357) -> (max value=w356:dbl, min value=w355:dbl)  [unwired: 2 out]
    n197 = Array Max & Min(array=w358) -> (max value=w354:dbl, min value=w353:dbl)  [unwired: 2 out]
    n198 = call "Attitude Control Write.vi"("pitch (x), roll (y), yaw (z)"=w370, "Attitude Control Handle In"=w371) -> ("Attitude Control Handle Out"=w369:T11)  [unwired: 8 in, 1 out]
    n199 = call "axis equal in labview.vi"("y min"=w353, "y max"=w354, "x min"=w355, "x max"=w356) -> ("yscale min"=w359:dbl, "yscale max"=w360:dbl, "xscale min"=w361:dbl, "xscale max"=w362:dbl)  [unwired: 4 in]
    n200 = property class="XYGraph (strict)"(reference=w363, "XScale.Maximum"=w362, "XScale.Minimum"=w361, "YScale.Maximum"=w360, "YScale.Minimum"=w359) -> ()  [unwired: 1 in, 2 out]
    n201 = Wait (ms)(milliseconds to wait=u32 20) -> ()  [unwired: 1 out]
    n202 = local read "stop"() -> (w390:bool)
  }
  n203 = call "Attitude Control Close.vi"("Attitude Control Handle"=w20) -> ()  [unwired: 10 in, 1 out]
